vi "VisChroma.vi"() -> ()   [LabVIEW 2018, in "AcPwrPlugins.lvlib" / "ChromaAcLoad.lvclass"]
uses:
  ChromaAcLoad.lvclass
  TypeDefs/MeasurementData.ctl
  TypeDefs/Measurements.ctl
  TypeDefs/MeasurementType.ctl
  <vilib>/Utility/error.llb/Error Cluster From Error Code.vi
  <vilib>/ErrorRing/Error Ring.xnode
  <userlib>/NIST/NISTErrorLib/NISTErrorLib.lvlib
  AcPwrPlugins.lvlib
panel:
  in  "Tab Control":enum32{"Chart", "XY Graph"}(tab)
  out "Chroma":waveform(dbl)[](graph)=[{"t0"=timestamp(3657200531.6397257 s since 1904-01-01), "dt"=1.0, "Y"=[46.19]}, {"t0"=timestamp(3657200531.6397257 s since 1904-01-01), "dt"=1.0, "Y"=[2.0]}, {"t0"=timestamp(3657200531.6397257 s since 1904-01-01), "dt"=1.0, "Y"=[60.0]}]
  in  "PlotYAxis":u32[](array[numeric])=[0, 1, 0] max=1
  out "Incorrect DataType?":bool
  out "Chroma's Internal Errors/Warnings":string="No Error"
  out "Current (A)":dbl(knob) scale=0.0..15.0
  out "Voltage (V)":dbl(knob) scale=0.0..100.0
  out "XY Graph":cluster{dbl[], dbl[]}(graph)={[0.02, 0.02, 0.02, 0.02, 0.02, 0.02, 0.02, 0.02, 0.1, 0.1, 0.1, 0.1, 0.1, 0.11, 0.2, 0.2, 0.2, 0.2, 0.2, 0.2, 0.3, 0.3, 0.3, 0.3, 0.3, 0.3, 0.3, 0.37, 0.4, 0.4, 0.4, 0.4, 0.4, 0.4, 0.48, 0.5, 0.5, 0.5, 0.5, 0.5, 0.5, 0.59, 0.6, 0.6, 0.6, 0.6, 0.6, 0.6, 0.6, 0.69, 0.69, 0.69, 0.69, 0.69, 0.69, 0.71, 0.79, 0.79, 0.79, 0.79, 0.79, 0.79, 0.89, 0.89, 0.89, 0.89, 0.89, 0.89, 0.89, 1.0, 1.0, 1.0, 1.0, 1.0, 1.0, 1.0, 1.1, 1.1, 1.1, 1.09, 1.09, 1.09, 1.1, 1.19, 1.19, 1.2, 1.2, 1.2, 1.2, 1.2, 1.29, 1.29, 1.29, 1.29, 1.29, 1.29, 1.29, 1.39, 1.39, 1.39, 1.39, 1.39, 1.39, 1.39, 1.4, 1.49, 1.49, 1.49, 1.49, 1.49, 1.49, 1.57, 1.59, 1.59, 1.59, 1.59, 1.59, 1.59, 1.69, 1.69, 1.69, 1.69, 1.69, 1.69, 1.69, 1.79, 1.79, 1.79, 1.79, 1.79, 1.79, 1.79, 1.89, 1.89, 1.89, 1.89, 1.89, 1.89, 1.89, 1.99, 1.99, 1.99, 1.99, 1.99, 1.99, 2.0, 2.09, 2.09, 2.09, 2.09, 2.09, 2.09, 2.13, 2.19, 2.19, 2.19, 2.19, 2.19, 2.19, 2.29, 2.29, 2.29, 2.29, 2.29, 2.29, 2.29, 2.29, 2.39, 2.39, 2.39, 2.39, 2.39, 2.39, 2.39, 2.49, 2.49, 2.49, 2.49, 2.49, 2.49, 2.51, 2.59, 2.59, 2.59, 2.59, 2.59, 2.59, 2.69, 2.69, 2.69, 2.69, 2.69, 2.69, 2.69, 2.79, 2.79, 2.79, 2.79, 2.79, 2.79, 2.79, 2.81, 2.89, 2.89, 2.89, 2.89, 2.89, 2.89, 2.89, 2.99, 2.99, 2.99, 2.99, 2.99, 2.99, 3.0, 3.09, 3.09, 3.09, 3.09, 3.09, 3.09, 3.1, 3.19, 3.19, 3.19, 3.19, 3.19, 3.19, 3.29, 3.29, 3.29, 3.29, 3.29, 3.29, 3.29, 3.39, 3.39, 3.39, 3.39, 3.39, 3.39, 3.39, 3.39, 3.49, 3.49, 3.49, 3.49, 3.49, 3.49, 3.49, 3.5, 3.59, 3.59, 3.59, 3.59, 3.59, 3.59, 3.6, 3.69, 3.69, 3.69, 3.69, 3.69, 3.69, 3.79, 3.79, 3.79, 3.79, 3.79, 3.79, 3.79, 3.89, 3.89, 3.89, 3.89, 3.89, 3.89, 3.89, 3.99, 3.99, 3.99, 3.99, 3.99, 3.99, 3.99], [42.02, 41.83, 42.15, 41.98, 41.52, 41.47, 41.64, 41.55, 41.51, 41.49, 41.46, 41.51, 41.41, 41.39, 41.42, 41.42, 41.41, 41.4, 41.29, 41.3, 41.32, 41.33, 41.32, 41.31, 41.32, 41.21, 41.21, 41.2, 41.2, 41.21, 41.22, 41.21, 41.1, 41.1, 41.09, 41.1, 41.09, 41.11, 41.1, 40.98, 40.99, 40.98, 40.98, 40.99, 40.99, 40.98, 40.98, 40.86, 40.86, 40.88, 40.87, 40.88, 40.87, 40.87, 40.74, 40.75, 40.75, 40.75, 40.73, 40.76, 40.63, 40.63, 40.62, 40.64, 40.64, 40.61, 40.64, 40.6, 40.5, 40.46, 40.5, 40.51, 40.5, 40.51, 40.37, 40.37, 40.37, 40.37, 40.37, 40.38, 40.37, 40.36, 40.22, 40.23, 40.23, 40.24, 40.23, 40.24, 40.1, 40.09, 40.07, 40.11, 40.09, 40.09, 40.11, 39.96, 39.96, 39.95, 39.96, 39.96, 39.96, 39.94, 39.81, 39.79, 39.79, 39.81, 39.8, 39.79, 39.79, 39.81, 39.65, 39.65, 39.65, 39.65, 39.64, 39.64, 39.65, 39.48, 39.48, 39.48, 39.48, 39.47, 39.48, 39.31, 39.31, 39.3, 39.31, 39.32, 39.31, 39.31, 39.14, 39.13, 39.13, 39.14, 39.13, 39.14, 39.13, 38.95, 38.95, 38.95, 38.94, 38.95, 38.95, 38.95, 38.75, 38.75, 38.76, 38.76, 38.75, 38.75, 38.75, 38.56, 38.56, 38.56, 38.56, 38.56, 38.55, 38.34, 38.34, 38.34, 38.33, 38.33, 38.34, 38.34, 38.11, 38.11, 38.1, 38.11, 38.12, 38.1, 38.11, 38.11, 37.87, 37.86, 37.86, 37.88, 37.86, 37.88, 37.86, 37.6, 37.61, 37.61, 37.61, 37.61, 37.61, 37.62, 37.33, 37.34, 37.33, 37.34, 37.34, 37.34, 37.04, 37.04, 37.05, 37.04, 37.06, 37.05, 37.04, 36.72, 36.72, 36.71, 36.72, 36.73, 36.72, 36.71, 36.72, 36.38, 36.37, 36.39, 36.37, 36.37, 36.38, 36.37, 36.0, 36.0, 35.99, 36.0, 35.99, 36.0, 35.99, 35.59, 35.59, 35.58, 35.58, 35.58, 35.58, 35.12, 35.12, 35.12, 35.13, 35.13, 35.13, 35.12, 34.6, 34.59, 34.59, 34.59, 34.59, 34.59, 34.59, 34.6, 33.97, 33.97, 33.98, 33.97, 33.98, 33.98, 33.98, 33.26, 33.27, 33.26, 33.26, 33.26, 33.26, 33.26, 33.26, 32.38, 32.39, 32.39, 32.37, 32.37, 32.39, 32.38, 31.25, 31.24, 31.25, 31.25, 31.25, 31.25, 29.64, 29.66, 29.66, 29.67, 29.65, 29.66, 29.66, 27.14, 27.15, 27.15, 27.15, 27.14, 27.14, 27.15, 17.86, 17.84]}
  in  "PluginName":string="AcPwr.Chroma0"
  out "ErrorArray":errorcluster[](array[cluster])
  in  "QueuName":string="CHROMADCVQ"
  in  "btnStop":bool
  in  "btnReset":bool
  in  "btnClear":bool
  # "0=Left Axis and 1=Right Axis"
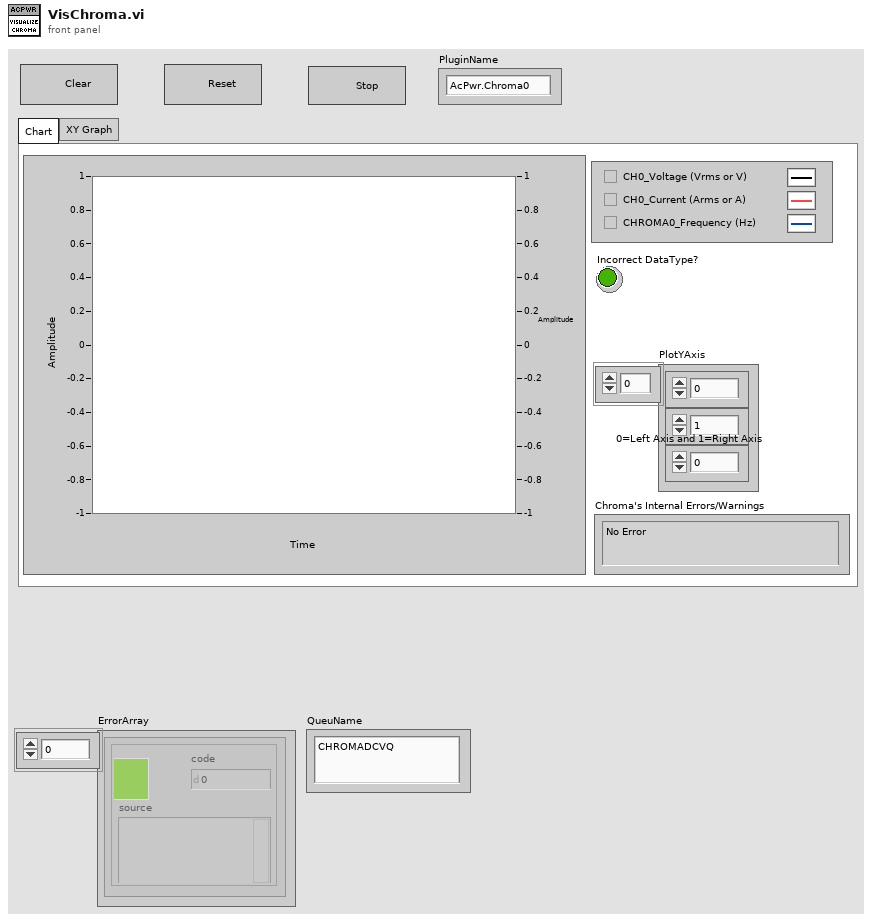
[diagram p1: front panel]
types:
  T1 = typedef "clBroadcastEvents.ctl" = cluster{"DidInit":refnum<user-event>, "StatusUpdate":refnum<user-event>, "ErrorReport":refnum<user-event>, "DidStop":refnum<user-event>, "PathToINI":refnum<user-event>, "Measurements":refnum<user-event>, "LoadConfigFile":refnum<user-event>, "GetSettings":refnum<user-event>, "SetSettings":refnum<user-event>, "GetType&ID":refnum<user-event>, "GotSettings":refnum<user-event>}
  T2 = typedef "AcPwrPlugins.lvlib/ChromaAcLoad.lvclass/MeasurementData.ctl" = cluster{"Time Stamp":timestamp, "Measurements":T3}
  T3 = typedef "AcPwrPlugins.lvlib/ChromaAcLoad.lvclass/Measurements.ctl" = cluster{"Handle":string, "Name":string, "Enabled":bool, "Measurement Value":dbl, "Hold Peak Current Measurement":bool, "btnMeasFetch":bool, "ProtectionStatusString":string, "Measurement Type":T4}[]
  T4 = typedef "AcPwrPlugins.lvlib/ChromaAcLoad.lvclass/MeasurementType.ctl" = enum16{"Voltage (Vrms or V)", "Current (Arms or A)", "Power (W)", "Peak Voltage (V)", "Peak Current (A)", "Peak Power (W)", "Frequency (Hz)", "Resistance (Ohms)", "Voltage Overshoot (V)", "Positive Peak Current (A)", "Voltage Undershoot (V)", "Negative Peak Current (A)", "Apparent Power (VA)", "Reacitive Power (VAR)", "Voltage THD", "Power Factor", "Current's Crest Factor"}
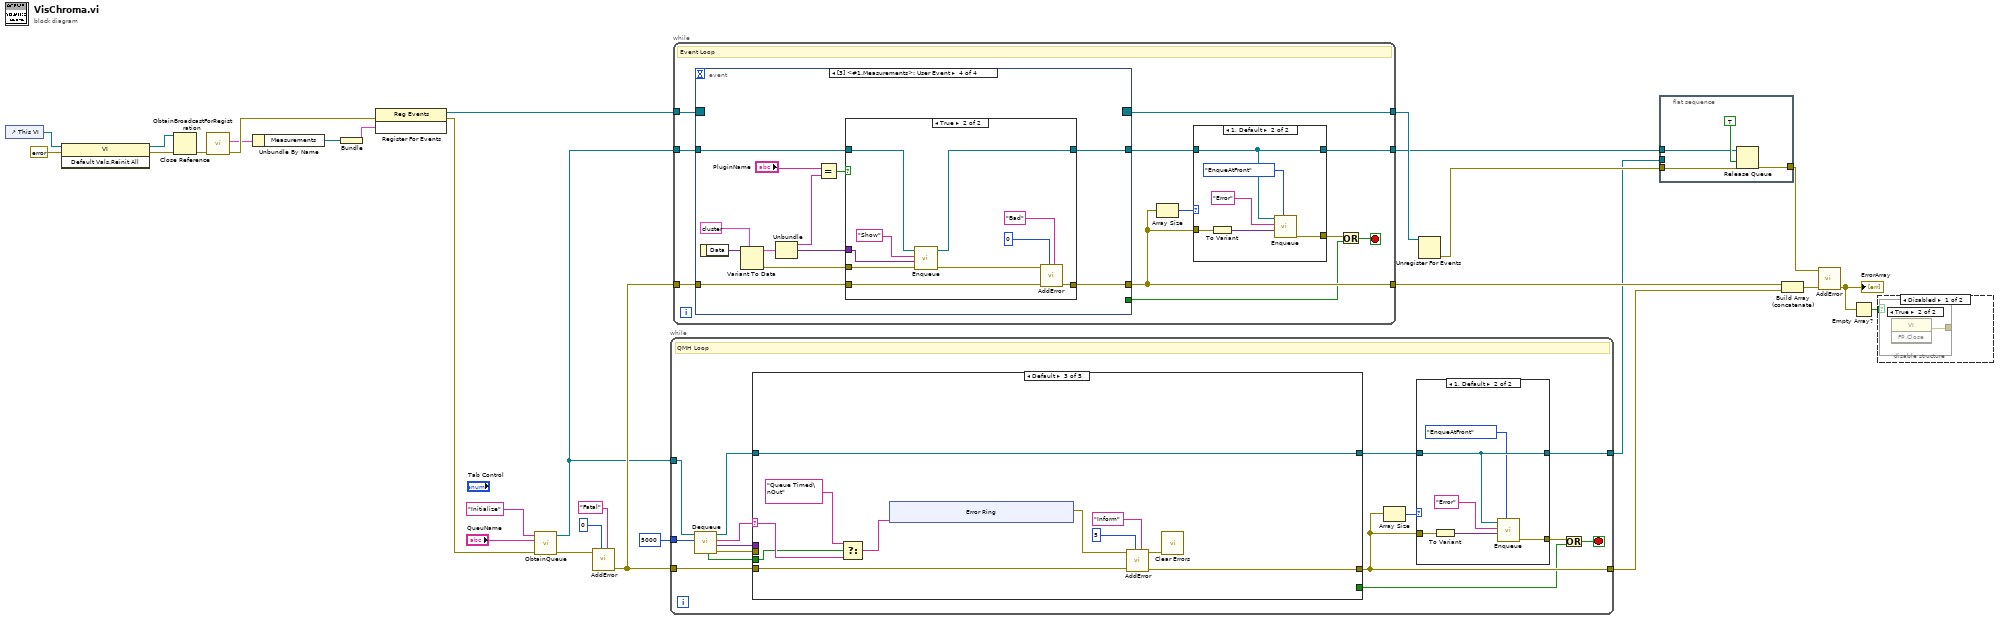
[diagram p0: block diagram]
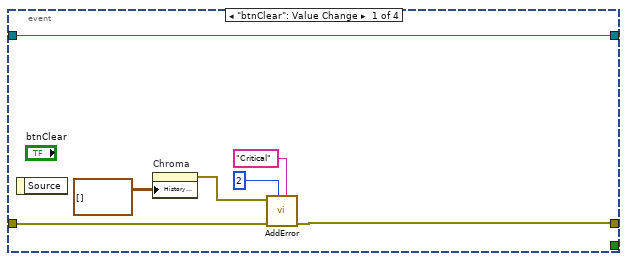
[diagram p5: hidden frame]
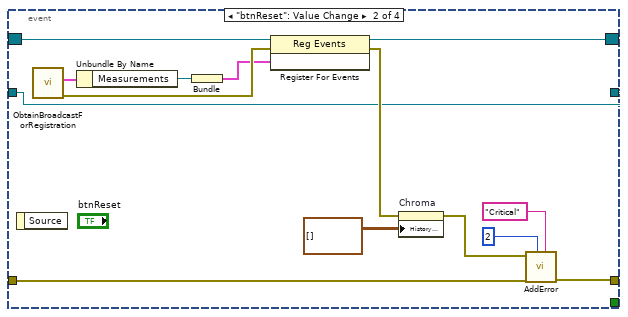
[diagram p6: hidden frame]
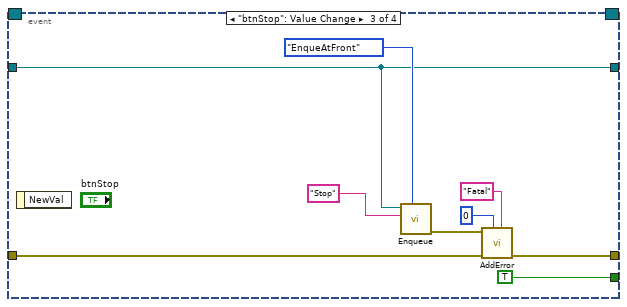
[diagram p7: hidden frame]
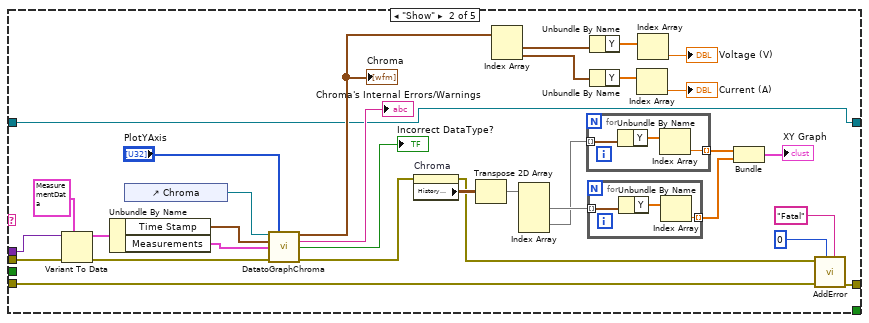
[diagram p11: hidden frame]
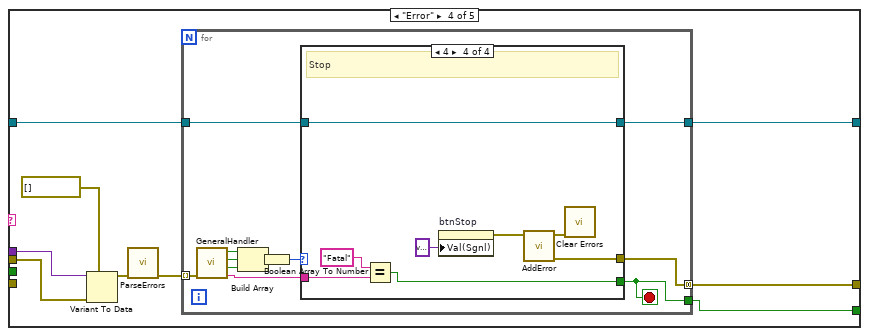
[diagram p12: hidden frame]
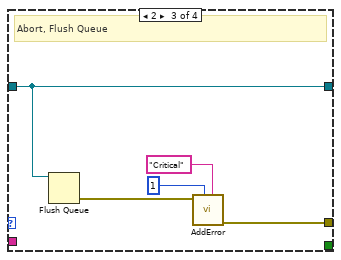
[diagram p15: hidden frame]
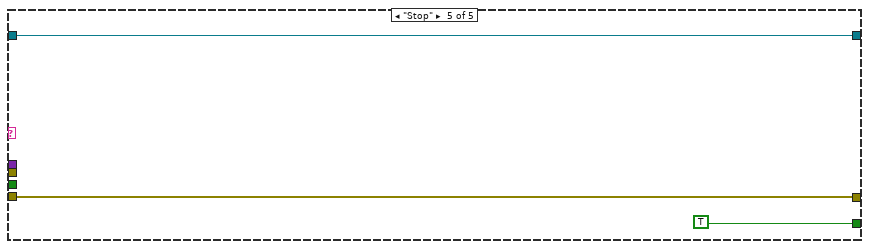
[diagram p16: hidden frame]
diagram:
  n1 = control-ref of="This VI"() -> (w19:refnum<vi>)
  n2 = invoke class="VI" method="Default Vals.Reinit All"(reference=w19, error in=errorcluster {"status"=FALSE, "code"=0, "source"=""} ("error in (no error)")) -> (reference out=w16:refnum<vi>, error out=w17:errorcluster)  [unwired: 1 in, 1 out]
  n3 = Close Reference(reference=w16, error in (no error)=w17) -> (error out=w15:errorcluster)
  n4 = call "ObtainBroadcastForRegistration.vi"("error in (no error)"=w15) -> ("error out"=w14:errorcluster, "clBroadcastEvents"=w13:T1)  [unwired: 9 in]
  n5 = Unbundle By Name(w13) -> ("Measurements"=w21:refnum<user-event>)
  n6 = Bundle("Measurements"=w21) -> (w20:cluster{"Measurements":refnum<user-event>})  [unwired: 1 in]
  n7 = register-events(error in=w14, w20) -> (reference out=w29:refnum<event-registration>, error out=w5:errorcluster)  [unwired: 1 in]
  n8 = call "ObtainQueue.vi"("error in (no error)"=w5, "ModuleName"="QueuName", "Initial Message"="Initialize" ("Message")) -> ("error out"=w8:errorcluster, "MessageQueue"=w4:refnum<queue>)  [unwired: 7 in]
  n9 = call <userlib>:"AddError.vi"("Severity"="Fatal", "Priority"=u8 0, "error in (no error)"=w8) -> ("ErrorArray"=w10:errorcluster[])  [unwired: 7 in, 1 out]
  n10 = while {
    tunnel: w10 -> [w42]
    tunnel: [w37] -> w9
    tunnel: w4 -> [w43]
    tunnel: [w35] -> w2
    tunnel: 5000 ("timeout in ms (-1)") -> [w33]
    stop <- w30 stop-if-true
    # "QMH Loop"
    n11 = call "Dequeue.vi"("timeout in ms (-1)"=w33, "MessageQueue"=w43) -> ("error out"=w40:errorcluster, "Message Data"=w44:variant, "Message"=w39:string, "MessageQueue"=w41:refnum<queue>, "timed out?"=w34:bool)  [unwired: 5 in]
    n12 = case shown="Default" w39 {
      selector: w39 -> [_ _ w95 _ _]
      tunnel: w44 -> [_ w63 _ w118 _]
      tunnel: w42 -> [w53 w83 w101 _ w146]
      tunnel: [w53 w85 w100 w114 w146] -> w37
      tunnel: [_ _ _ w113 TRUE] -> w31
      tunnel: w41 -> [w52 w54 w96 w112 w145]
      tunnel: w40 -> [_ w55 _ w111 _]
      tunnel: [w52 w54 w96 w110 w145] -> w38
      tunnel: w34 -> [_ _ w92 _ _]
      frame "Initialize" {
      }
      frame "Show" {
        n13 = Variant To Data(error in=w55, type=T2 {"Time Stamp"=timestamp(0 s since 1904-01-01), "Measurements"=[]} ("MeasurementData"), Variant=w63) -> (data=w61:T2, error out=w62:errorcluster)
        n14 = Unbundle By Name(w61) -> ("Time Stamp"=w60:timestamp, "Measurements"=w59:T3)
        n15 = control-ref of="Chroma"() -> (w84:refnum<vi>)
        n16 = call "DatatoGraphChroma.vi"("WaveformChartReference"=w84, "PlotYScale"="PlotYAxis", "Time Stamp"=w60, "Measurements"=w59, "error in (no error)"=w62) -> ("WaveformArray"=w70:waveform(dbl)[], "OutputString"=→"Chroma's Internal Errors/Warnings":string, "Incorrect DataType?"=→"Incorrect DataType?":bool, "error out"=w78:errorcluster)  [unwired: 7 in]
        "Chroma" <- w70
        n17 = property on="Chroma" class="WFChart (strict)"(error in=w78) -> (error out=w57:errorcluster, "History Data"=w76:waveform(dbl)[][])  [unwired: 1 in, 1 out]
        n18 = Transpose 2D Array(2D array=w76) -> (transposed array=w77:waveform(dbl)[][])
        n19 = Index Array(array=w70) -> (element #1=w69:waveform(dbl), element #2=w68:waveform(dbl))  [unwired: 2 in]
        n20 = Index Array(array=w77) -> (element #1=w73:waveform(dbl)[], element #2=w72:waveform(dbl)[])  [unwired: 4 in]
        n21 = for {
          tunnel: w72 -> [w91] mode=indexing
          tunnel: [w89] -> w74 mode=indexing
          n22 = Unbundle By Name(w91) -> ("Y"=w90:dbl[])
          n23 = Index Array(array=w90) -> (element=w89:dbl)  [unwired: 1 in]
        }
        n24 = for {
          tunnel: w73 -> [w88] mode=indexing
          tunnel: [w86] -> w75 mode=indexing
          n25 = Unbundle By Name(w88) -> ("Y"=w87:dbl[])
          n26 = Index Array(array=w87) -> (element=w86:dbl)  [unwired: 1 in]
        }
        n27 = Unbundle By Name(w69) -> ("Y"=w67:dbl[])
        n28 = Unbundle By Name(w68) -> ("Y"=w66:dbl[])
        n29 = Index Array(array=w66) -> (element=→"Current (A)":dbl)  [unwired: 1 in]
        n30 = Index Array(array=w67) -> (element=→"Voltage (V)":dbl)  [unwired: 1 in]
        n31 = Bundle(w74, w75) -> (→"XY Graph":cluster{dbl[], dbl[]})  [unwired: 1 in]
        n32 = call <userlib>:"AddError.vi"("Severity"="Fatal" ("String"), "Priority"=u8 0, "ErrorArray"=w83, "error in (no error)"=w57) -> ("ErrorArray"=w85:errorcluster[])  [unwired: 6 in, 1 out]
      }
      frame Default {
        n33 = Select(t="Queue Timed\nOut", s=w92, f=w95) -> (s? t:f=w94:string)
        n34 = xnode "Error Ring"("parameter 0"=w94) -> ("error out"=w102:errorcluster)
        n35 = call <userlib>:"AddError.vi"("Severity"="Inform" ("String"), "Priority"=u8 5, "ErrorArray"=w101, "error in (no error)"=w102) -> ("ErrorArray"=w100:errorcluster[], "error out"=w99:errorcluster)  [unwired: 6 in]
        n36 = call <vilib>:"Clear Errors.vi"("error in (no error)"=w99) -> ()  [unwired: 5 in, 2 out]
      }
      frame "Error" {
        n37 = Variant To Data(error in=w111, type=errorcluster[] [], Variant=w118) -> (data=w116:errorcluster[])  [unwired: 1 out]
        n38 = call <userlib>:"ParseErrors.vi"("ErrorArray"=w116) -> ("ErrorArray"=w115:errorcluster[])  [unwired: 8 in, 2 out]
        n39 = for {
          tunnel: w115 -> [w129] mode=indexing
          tunnel: [w123] -> w114 mode=concatenating
          tunnel: [w121] -> w113
          tunnel: w112 -> [w120]
          tunnel: [w119] -> w110
          stop <- w121 stop-if-true
          n40 = call <userlib>:"GeneralHandler.vi"("error in (no error)"=w129) -> ("Severity"=w122:string, "Stop"=w126:bool, "Abort"=w127:bool, "Continue"=w128:bool)  [unwired: 7 in]
          n41 = Build Array(w128, w127, w126) -> (w125:bool[])
          n42 = Boolean Array To Number(Boolean array=w125) -> (number=w124:u32)
          n43 = case shown="4" w124 {
            tunnel: [_ _ w136 w144] -> w123
            tunnel: w122 -> [_ _ _ w142]
            tunnel: [_ _ _ w140] -> w121
            tunnel: w120 -> [w130 w131 w132 w137]
            tunnel: [w130 w131 w132 w137] -> w119
            frame 0, Default {
              # "No Dialog"
            }
            frame 1 {
              # "Continue"
            }
            frame 2 {
              # "Abort, Flush Queue"
              n44 = Flush Queue(queue=w132) -> (error out=w135:errorcluster)  [unwired: 1 in, 2 out]
              n45 = call <userlib>:"AddError.vi"("Severity"="Critical" ("String"), "Priority"=u8 1, "error in (no error)"=w135) -> ("ErrorArray"=w136:errorcluster[])  [unwired: 7 in, 1 out]
            }
            frame 4 {
              # "Stop"
              n46 = Equal?(x="Fatal", y=w142) -> (x = y?=w140:bool)
              n47 = property on="btnStop" class="Bool"("Val(Sgnl)"=variant ("Value (Signaling)")) -> (error out=w139:errorcluster)  [unwired: 2 in, 1 out]
              n48 = call <userlib>:"AddError.vi"("error in (no error)"=w139) -> ("ErrorArray"=w144:errorcluster[], "error out"=w143:errorcluster)  [unwired: 9 in]
              n49 = call <vilib>:"Clear Errors.vi"("error in (no error)"=w143) -> ()  [unwired: 5 in, 2 out]
            }
          }
        }
      }
      frame "Stop" {
      }
    }
    n50 = Array Size(array=w37) -> (size(s)=w36:i32)
    n51 = case shown="1, Default" w36 {
      tunnel: [_ w46] -> w32
      tunnel: w37 -> [_ w51]
      tunnel: w38 -> [w45 w48]
      tunnel: [w45 w48] -> w35
      frame 0 {
      }
      frame 1, Default {
        n52 = To Variant(anything=w51) -> (Variant=w50:variant)
        n53 = call "Enqueue.vi"("EnqueType (Enque)"=enum16{"LossyEnque", "EnqueAtFront", "Enque"}."EnqueAtFront", "Message Data"=w50, "Message"="Error", "MessageQueue"=w48) -> ("error out"=w46:errorcluster)  [unwired: 6 in, 1 out]
      }
    }
    n54 = Or(x=w32, y=w31) -> (x .or. y?=w30:bool)
  }
  n55 = while {
    tunnel: w29 -> [w158]
    tunnel: [w153] -> w27
    tunnel: [w157] -> w28
    tunnel: w10 -> [w156]
    tunnel: w4 -> [w155]
    tunnel: [w151] -> w3
    stop <- w148 stop-if-true
    # "Event Loop"
    n56 = event shown="[3] <#1.Measurements>: User Event" {
      selector: w158 -> [_ w186 _ _]
      dyn-events: [_ w185 _ _] -> w157
      timeout: _ -> [_ _ _ _]
      tunnel: [_ _ TRUE _] -> w150
      tunnel: [w169 w180 w195 w207] -> w153
      tunnel: w156 -> [w170 w181 w189 w205]
      tunnel: w155 -> [w166 w173 w187 w197]
      tunnel: [w166 w173 w187 w196] -> w152
      event "btnClear": Value Change {
        n57 = event-data() -> ()  [unwired: 1 in, 1 out]
        n58 = property on="Chroma" class="WFChart (strict)"("History Data"=waveform(dbl)[][] []) -> (error out=w168:errorcluster)  [unwired: 2 in, 1 out]
        n59 = call <userlib>:"AddError.vi"("Severity"="Critical", "Priority"=u8 2, "ErrorArray"=w170, "error in (no error)"=w168) -> ("ErrorArray"=w169:errorcluster[])  [unwired: 6 in, 1 out]
      }
      event "btnReset": Value Change {
        n60 = event-data() -> ()  [unwired: 1 in, 1 out]
        n61 = call "ObtainBroadcastForRegistration.vi"() -> ("error out"=w182:errorcluster, "clBroadcastEvents"=w183:T1)  [unwired: 10 in]
        n62 = Unbundle By Name(w183) -> ("Measurements"=w184:refnum<user-event>)
        n63 = Bundle("Measurements"=w184) -> (w174:cluster{"Measurements":refnum<user-event>})  [unwired: 1 in]
        n64 = register-events(reference=w186, error in=w182, w174) -> (reference out=w185:refnum<event-registration>, error out=w176:errorcluster)
        n65 = property on="Chroma" class="WFChart (strict)"(error in=w176, "History Data"=waveform(dbl)[][] []) -> (error out=w175:errorcluster)  [unwired: 1 in, 1 out]
        n66 = call <userlib>:"AddError.vi"("Severity"="Critical", "Priority"=u8 2, "ErrorArray"=w181, "error in (no error)"=w175) -> ("ErrorArray"=w180:errorcluster[])  [unwired: 6 in, 1 out]
      }
      event "btnStop": Value Change {
        n67 = event-data() -> ()  [unwired: 1 in, 1 out]
        n68 = call "Enqueue.vi"("EnqueType (Enque)"=enum16{"LossyEnque", "EnqueAtFront", "Enque"}."EnqueAtFront", "Message"="Stop", "MessageQueue"=w187) -> ("error out"=w190:errorcluster)  [unwired: 7 in, 1 out]
        n69 = call <userlib>:"AddError.vi"("Severity"="Fatal" ("String"), "Priority"=u8 0, "ErrorArray"=w189, "error in (no error)"=w190) -> ("ErrorArray"=w195:errorcluster[])  [unwired: 6 in, 1 out]
      }
      event User Event {
        n70 = event-data() -> ("Data"=w201:variant)  [unwired: 1 in]
        n71 = Variant To Data(type=cluster{string, "Data":variant, string} {"", "Data"=variant, ""}, Variant=w201) -> (data=w204:cluster{string, "Data":variant, string}, error out=w202:errorcluster)  [unwired: 1 in]
        n72 = Unbundle(w204) -> (w203:string, "Data"=w199:variant)  [unwired: 1 out]
        n73 = Equal?(x="PluginName", y=w203) -> (x = y?=w206:bool)
        n74 = case shown="True" w206 {
          tunnel: [w209 w216] -> w207
          tunnel: w205 -> [w209 w217]
          tunnel: w202 -> [_ w212]
          tunnel: w199 -> [_ w214]
          tunnel: w197 -> [w208 w211]
          tunnel: [w208 w210] -> w196
          frame False {
          }
          frame True {
            n75 = call "Enqueue.vi"("error in (no error)"=w212, "Message Data"=w214, "Message"="Show", "MessageQueue"=w211) -> ("error out"=w213:errorcluster, "MessageQueue"=w210:refnum<queue>)  [unwired: 6 in]
            n76 = call <userlib>:"AddError.vi"("Severity"="Bad" ("String"), "Priority"=u8 0, "ErrorArray"=w217, "error in (no error)"=w213) -> ("ErrorArray"=w216:errorcluster[])  [unwired: 6 in, 1 out]
          }
        }
      }
    }
    n77 = Array Size(array=w153) -> (size(s)=w154:i32)
    n78 = case shown="1, Default" w154 {
      tunnel: [_ w160] -> w149
      tunnel: w153 -> [_ w165]
      tunnel: w152 -> [w159 w162]
      tunnel: [w159 w162] -> w151
      frame 0 {
      }
      frame 1, Default {
        n79 = To Variant(anything=w165) -> (Variant=w164:variant)
        n80 = call "Enqueue.vi"("EnqueType (Enque)"=enum16{"LossyEnque", "EnqueAtFront", "Enque"}."EnqueAtFront", "Message Data"=w164, "Message"="Error", "MessageQueue"=w162) -> ("error out"=w160:errorcluster)  [unwired: 6 in, 1 out]
      }
    }
    n81 = Or(x=w149, y=w150) -> (x .or. y?=w148:bool)
  }
  n82 = Unregister For Events(event registration refnum=w28) -> (error out=w26:errorcluster)  [unwired: 1 in]
  n83 = flat-sequence {
    tunnel: w26 -> [w220]
    tunnel: [w223] -> w24
    tunnel: w3 -> [w221]
    tunnel: w2 -> [_]
    frame #0 {
      n84 = Release Queue(queue=w221, force destroy? (F)=TRUE, error in (no error)=w220) -> (error out=w223:errorcluster)  [unwired: 2 out]
    }
  }
  n85 = Build Array (concatenate)(w27, w9) -> (w25:errorcluster[])
  n86 = call <userlib>:"AddError.vi"("ErrorArray"=w25, "error in (no error)"=w24) -> ("ErrorArray"=w23:errorcluster[])  [unwired: 8 in, 1 out]
  "ErrorArray" <- w23
  n87 = Empty Array?(array=w23) -> (empty?=w22:bool)
  n88 = disable-structure shown="Disabled" {
    disable-tunnel: w22 -> [w224 _]
    frame Disabled {
      n89 = case shown="True" w224 {
        tunnel: [_ w225] -> _
        frame False {
        }
        frame True {
          n90 = invoke class="VI" method="FP.Close"() -> (error out=w225:errorcluster)  [unwired: 3 in, 2 out]
        }
      }
    }
    frame Enabled {
    }
  }
